vi "Selet PCBs.vi"(0 "data in":T11, 1 "Programming Data":T6, 5 "Dongle Fitted event Refnum in":T1, 7 "Edit VI":refnum<vi>, 11 "error in":errorcluster) -> (4 "data out":T11, 6 "Back":bool, 8 "Dongle fitted":bool, 15 "error out":errorcluster)   [LabVIEW 2013, in "Manipulate IPF.lvlib"]
uses:
  Manipulate IPF.lvlib
  3013/code/Modules/GUI/GUI_5/subPanels/edit/type_def/data.ctl
  3013/code/Modules/Configuration/type_def/Scan Params.ctl
  3013/code/Modules/Configuration/type_def/Profile Resolution.ctl
  3013/code/Modules/Preprocess Data/type_def/direction.ctl
  3013/code/Modules/Inspection/Data/Panel_class/type_def/Config File data.ctl
  3013/code/Modules/Inspection/type_def/Pos and Rot.ctl
  3013/code/Modules/Inspection/Data/PCB_class/type_def/PCB Params.ctl
  3013/code/Modules/Inspection/Data/Panel_class/type_def/BarCode Params.ctl
  3013/code/Modules/Barcode Reader/type_def/id.ctl
  3013/code/Modules/Inspection/Data/Panel_class/type_def/inspection data.ctl
  3013/code/Modules/Inspection/type_def/Range Limits.ctl
  type_def/but_back.ctl
  type_def/but_continue.ctl
  type_def/files.ctl
  type_def/PCB List.ctl
  type_def/Dongle fitted event refnum.ctl
  Pack Data/type_def/file types.ctl
  <vilib>/Utility/cursorutil.llb/Set Cursor (Icon Pict).vi
  3013/code/Modules/Barcode Reader/Barcode Reader.lvlib
  3013/code/Modules/Inspection/Inspection.lvlib
  3013/code/Modules/Inspection/Data/PCB_class/PCB.lvclass
  a3Di APG.lvlib
  3013/code/Modules/Inspection/Data/Panel_class/Panel.lvclass
  Pack Data/Pack Files.lvlib
  3013/code/Modules/Configuration/Config.lvlib
  3013/code/Modules/Preprocess Data/PreProcess.lvlib
  3013/code/Modules/GUI/GUI_5/subPanels/edit/edit.lvlib
panel:
  out "Within outline":bool
  out "XY":cluster{"X":dbl, "Y":dbl}
  out "PCB Name":string
  in  "PCB List":T2 {"gui"."PCB Params"."Pos & Rot"."Y" format="%#_8g"; "gui"."PCB Params"."Pos & Rot"."X" format="%#_8g"}
  out "XY Graph":cluster{"X Out":dbl[], "Y Out":dbl[]}[](graph)
  in  "Continue Button":T9
  in  "Back Button":T10
  # "Select PCBs"
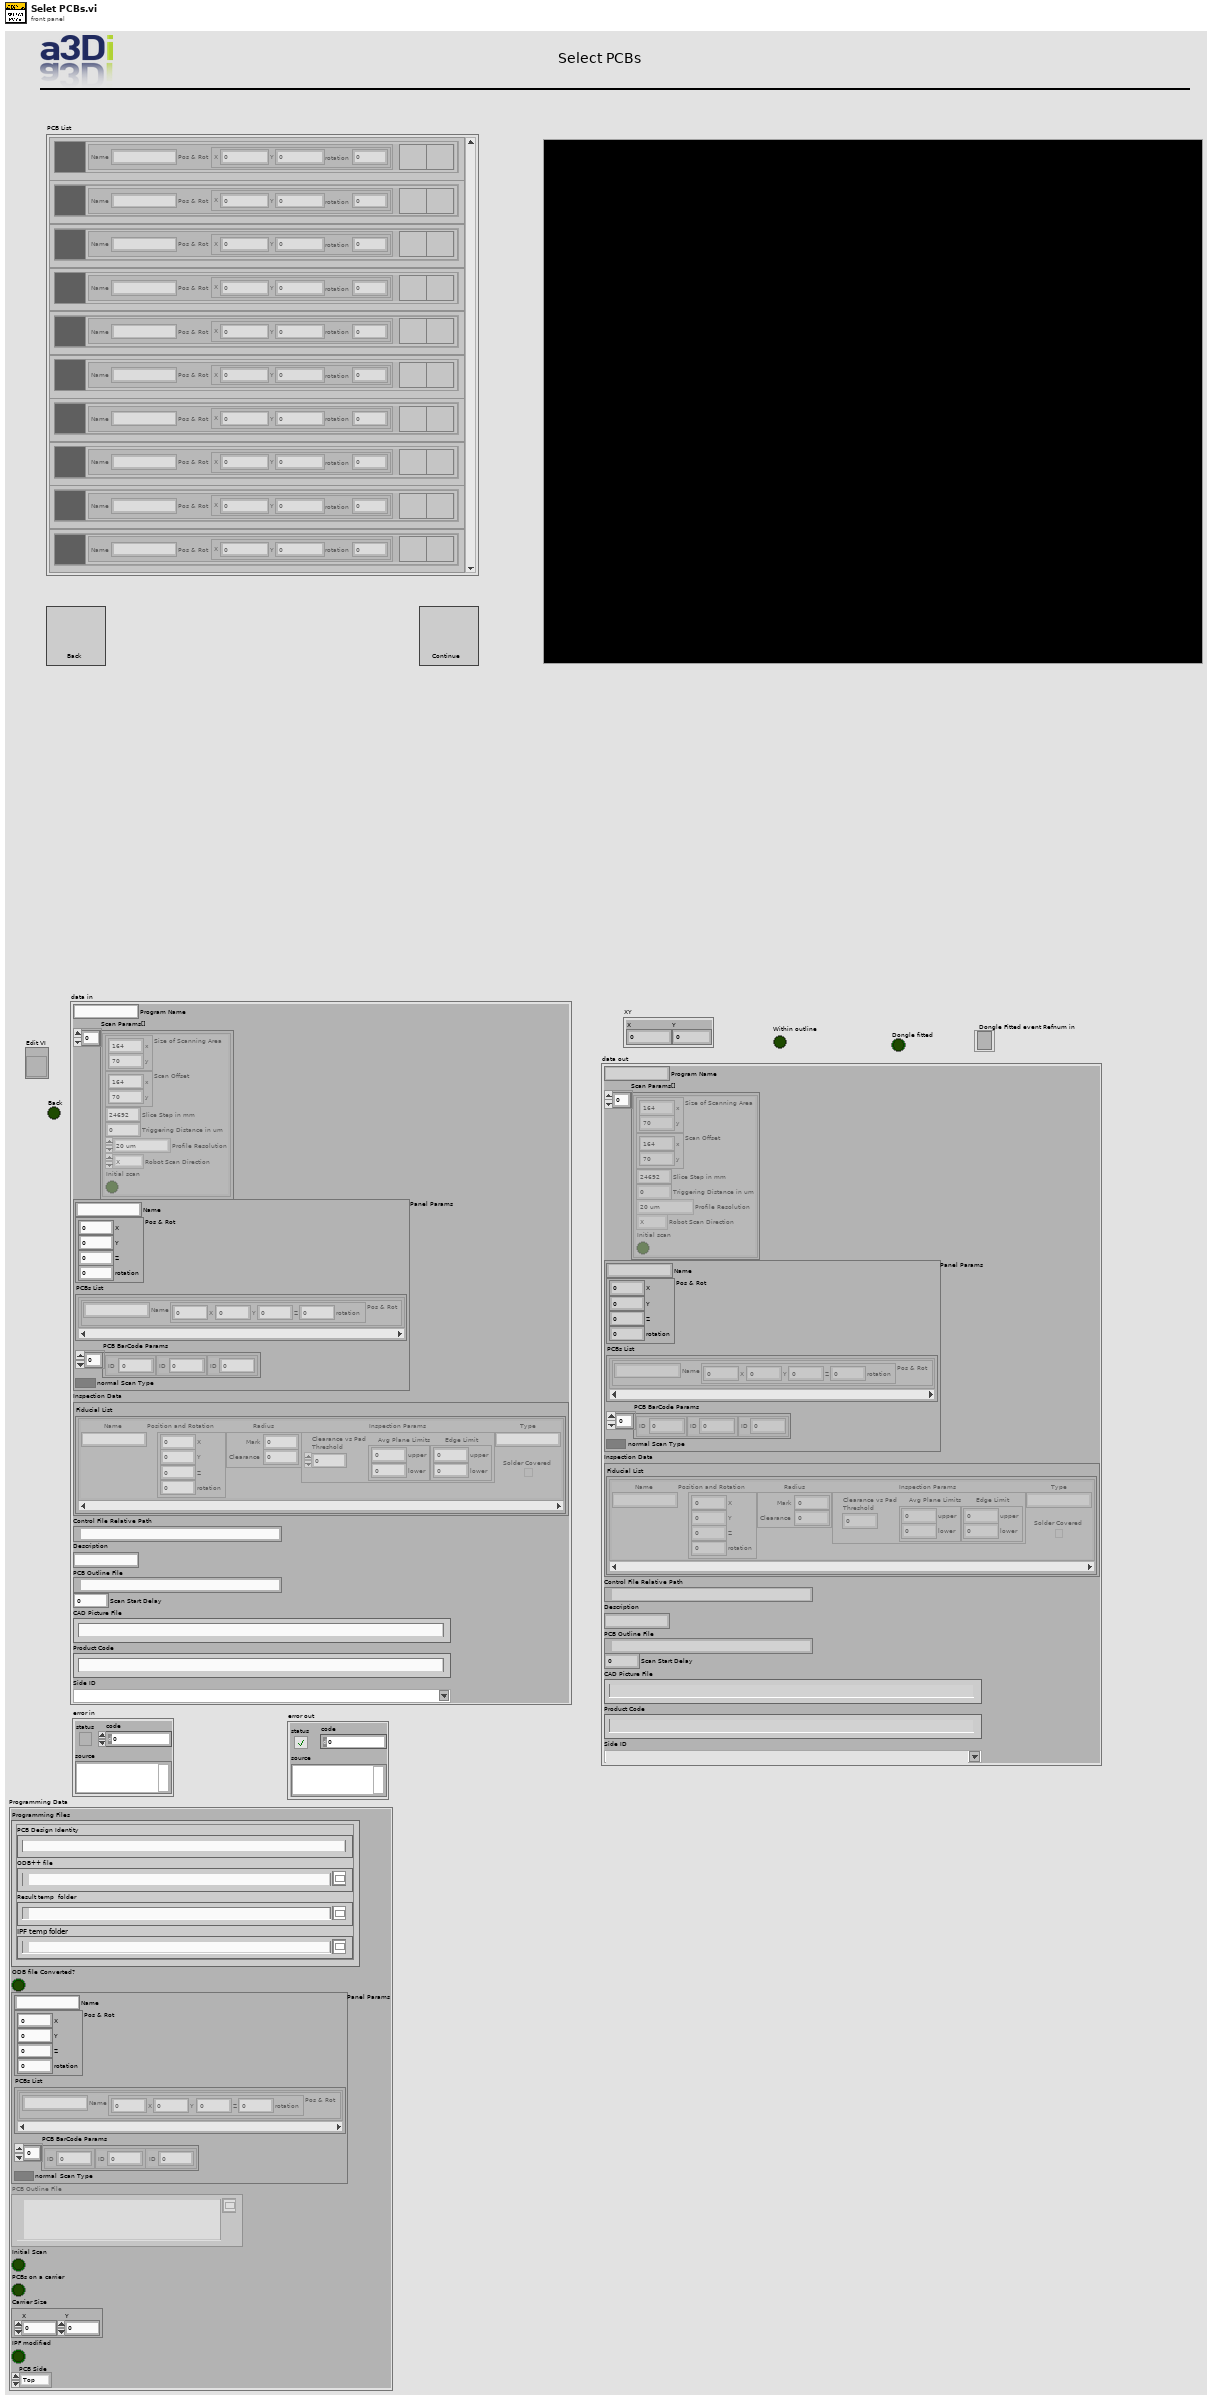
[diagram p1: front panel]
types:
  T1 = typedef "Dongle fitted event refnum.ctl" = refnum<event-registration>
  T2 = typedef "Manipulate IPF.lvlib/PCB List.ctl" = cluster{"Color Box":u32, "gui":cluster{"PCB Params":T3, "Barcode\nReader":cluster{"ID":T5}, "insert":bool, "delete":bool}}[]
  T3 = typedef "Inspection.lvlib/PCB.lvclass/PCB Params.ctl" = cluster{"Name":string, "Pos & Rot":T4}
  T4 = typedef "Inspection.lvlib/Pos and Rot.ctl" = cluster{"X":dbl, "Y":dbl, "Z":dbl, "rotation":dbl}
  T5 = typedef "Barcode Reader.lvlib/id.ctl" = u8
  T6 = typedef "a3Di APG.lvlib/files.ctl" = cluster{"Programming Files":cluster{"PCB Design Identity":string, "ODB++ file":path, "Result temp  folder":path, "IPF temp folder":path}, "ODB file Converted?":bool, "Panel Params":T7, "PCB Outline File":path, "Initial Scan":bool, "PCBs on a carrier":bool, "Carrier Size":cluster{"X":dbl, "Y":dbl}, "IPF modified":bool, "PCB Side":enum16{"Top", "Bottom"}}
  T7 = typedef "Inspection.lvlib/Panel.lvclass/Config File data.ctl" = cluster{"Name":string, "Pos & Rot":T4, "PCBs List":cluster{"PCB Params":T3}[], "PCB BarCode Params":T8[], "Scan Type":bool}
  T8 = typedef "Inspection.lvlib/Panel.lvclass/BarCode Params.ctl" = cluster{"ID":T5}
  T9 = typedef "but_continue.ctl" = bool
  T10 = typedef "a3Di APG.lvlib/but_back.ctl" = bool
  T11 = typedef "GUI.lvlib/subPanel.lvlib/edit.lvlib/data.ctl" = cluster{"Program Name":string, "Scan Params[]":T12[], "Panel Params":T7, "Inspection Data":T15, "Control File Relative Path":path, "Description":string, "PCB Outline File":path, "Scan Start Delay":dbl, "CAD Picture File":string, "Product Code":string, "Side ID":string}
  T12 = typedef "Config.lvlib/Scan Params.ctl" = cluster{"Size of Scanning Area":cluster{"x":dbl, "y":dbl}, "Scan Offset":cluster{"x":dbl, "y":dbl}, "Slice Step in mm":dbl, "Triggering Distance in mm":dbl, "Triggering Distance in um":dbl, "Profile Resolution":T13, "Version":string, "Robot Scan Direction":T14, "Initial scan":bool}
  T13 = typedef "Config.lvlib/Profile Resolution.ctl" = enum8{"20 um", "40 um"}
  T14 = typedef "PreProcess.lvlib/direction.ctl" = enum8{"X", "Y"}
  T15 = typedef "Inspection.lvlib/Panel.lvclass/inspection data.ctl" = cluster{"Fiducial List":cluster{"Name":string, "Position and Rotation":T4, "Radius":cluster{"Mark":dbl, "Clearance":dbl}, "Inspection Params":cluster{"Clearance vs Pad\nThreshold":dbl, "Avg Plane Limits":T16, "Edge Limit":T16}, "Type":string, "Solder Covered":bool}[]}
  T16 = typedef "Inspection.lvlib/Range Limits.ctl" = cluster{"upper":sgl, "lower":sgl}
  T17 = enum16{"Initialisaion", "Wait for user input", "exit"}
  T18 = cluster{"Plot colour":u32, "gui":cluster{"PCB Params":T3, "Barcode\nReader":cluster{"ID":T5}, "insert":bool, "delete":bool}}
  T19 = enum32{"Invalid", "Standard", "Closed", "Hidden", "Minimized", "Maximized"}
  T20 = typedef "Pack Files.lvlib/file types.ctl" = enum16{"ODB", "TCF", "CAD Outline", "Config", "Inspection Prog", "a3Di-bin", "Results", "CAD Labels", "CAD Pads", "calScan_fid", "calScan_cal-tab", "PCB_SerialNumber", "CAD_Assembly", "Version", "Old Results", "CAD Picture", "Old TCF"}
  T21 = enum8{"Enabled", "Disabled", "Disabled and Grayed Out"}
  T22 = cluster{"Plot colour":u32, "gui":cluster{"PCB Params":T3, "Barcode\nReader":cluster{"ID":T5}, "insert":bool, "delete":bool}}[]
  T23 = cluster{"Data":cluster{"X Out":dbl[], "Y Out":dbl[]}, "Name":string}[]
  T24 = cluster{"Color Box":bool, "gui":cluster{"PCB Params":cluster{"Name":bool, "Pos & Rot":cluster{"X":bool, "Y":bool, "Z":bool, "rotation":bool}}, "Barcode\nReader":cluster{"ID":bool}, "insert":bool, "delete":bool}}[]
  T25 = cluster{"Color Box":u32, "gui":cluster{"PCB Params":T3, "Barcode\nReader":cluster{"ID":T5}, "insert":bool, "delete":bool}}
  T26 = typedef "LVPoint32TypeDef.ctl" = cluster{"Horizontal":i32, "Vertical":i32}
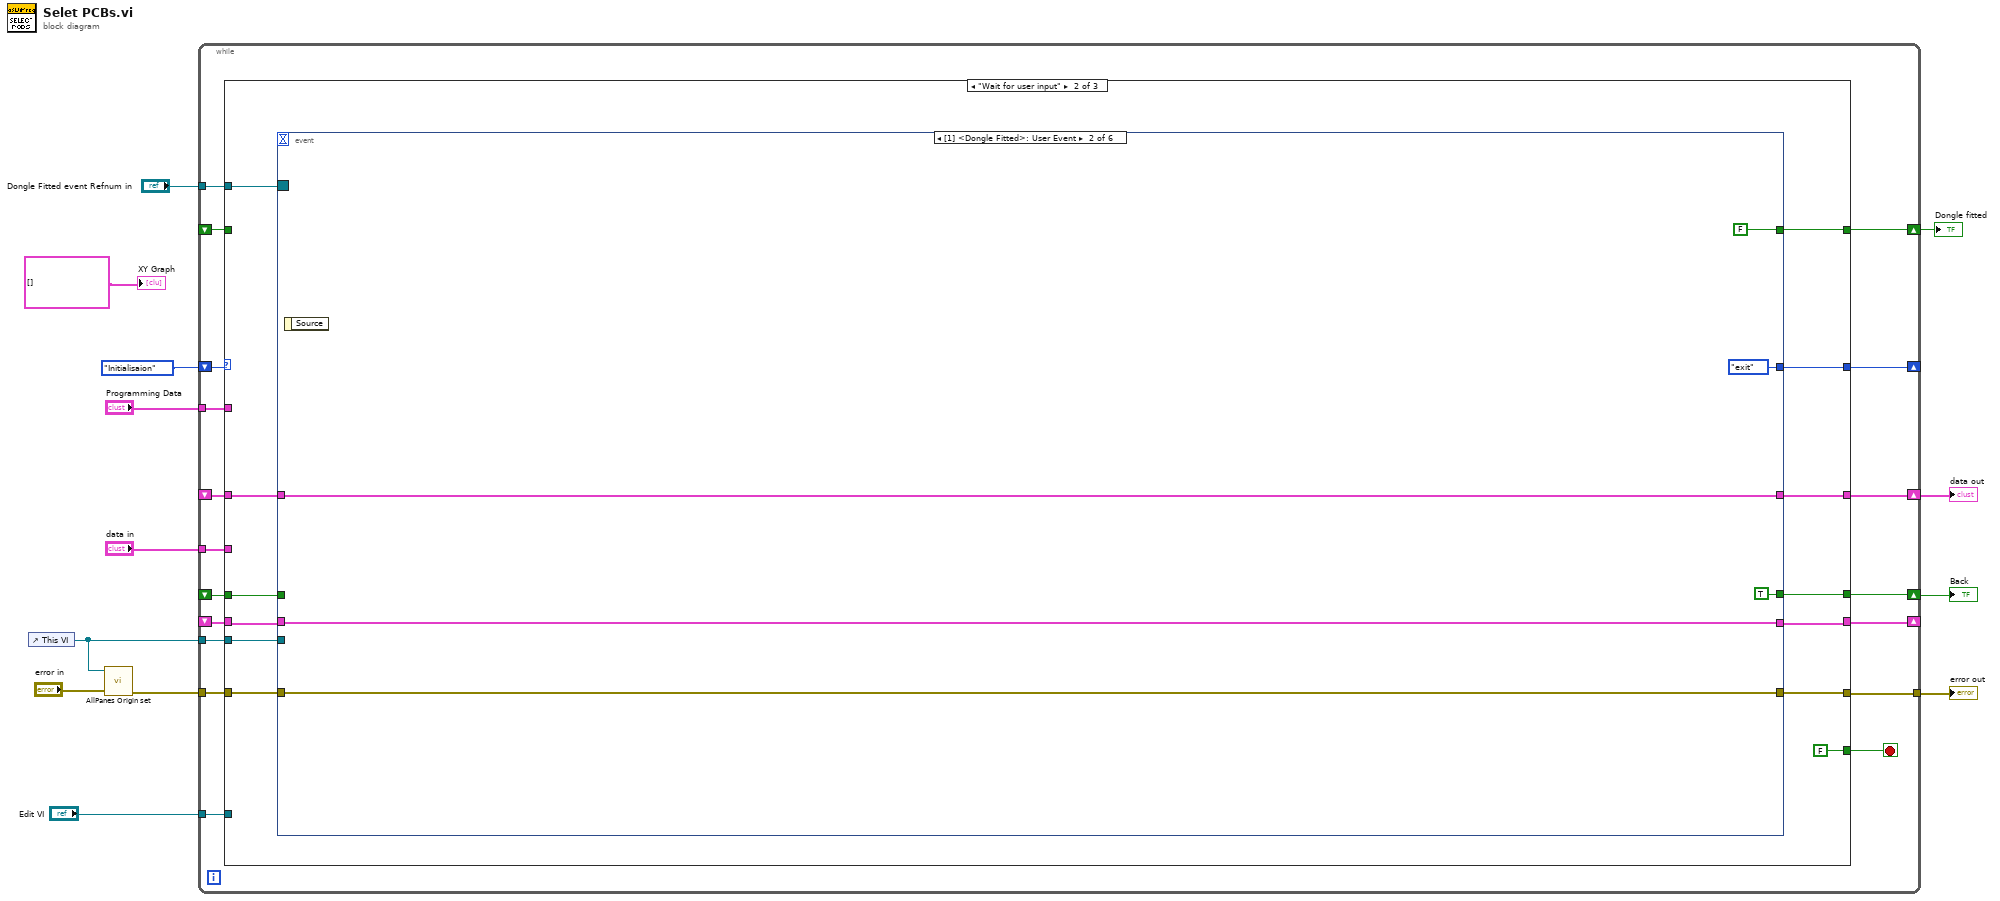
[diagram p0: block diagram]
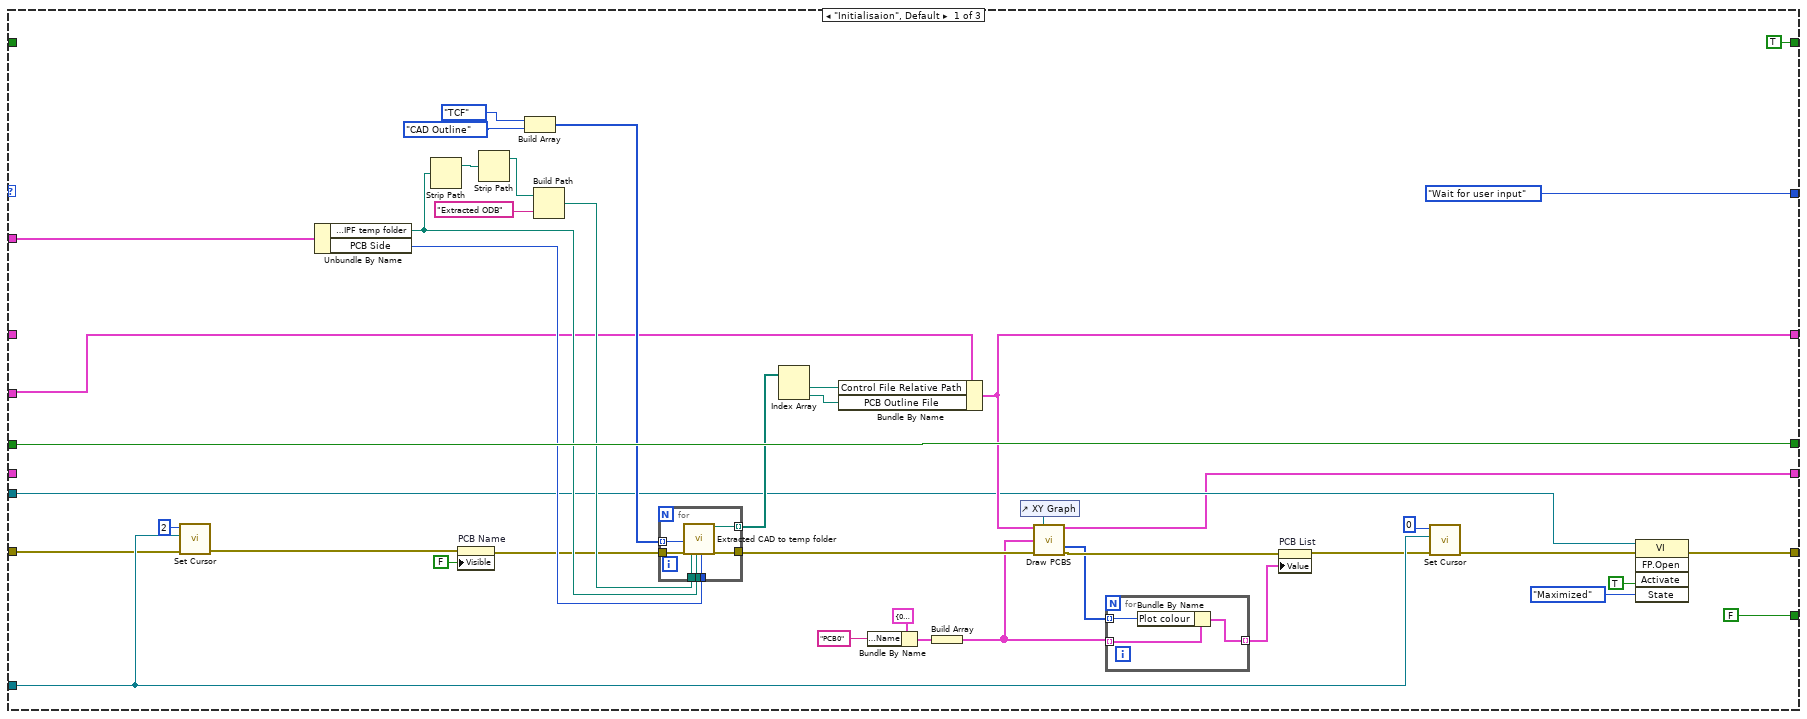
[diagram p2: hidden frame]
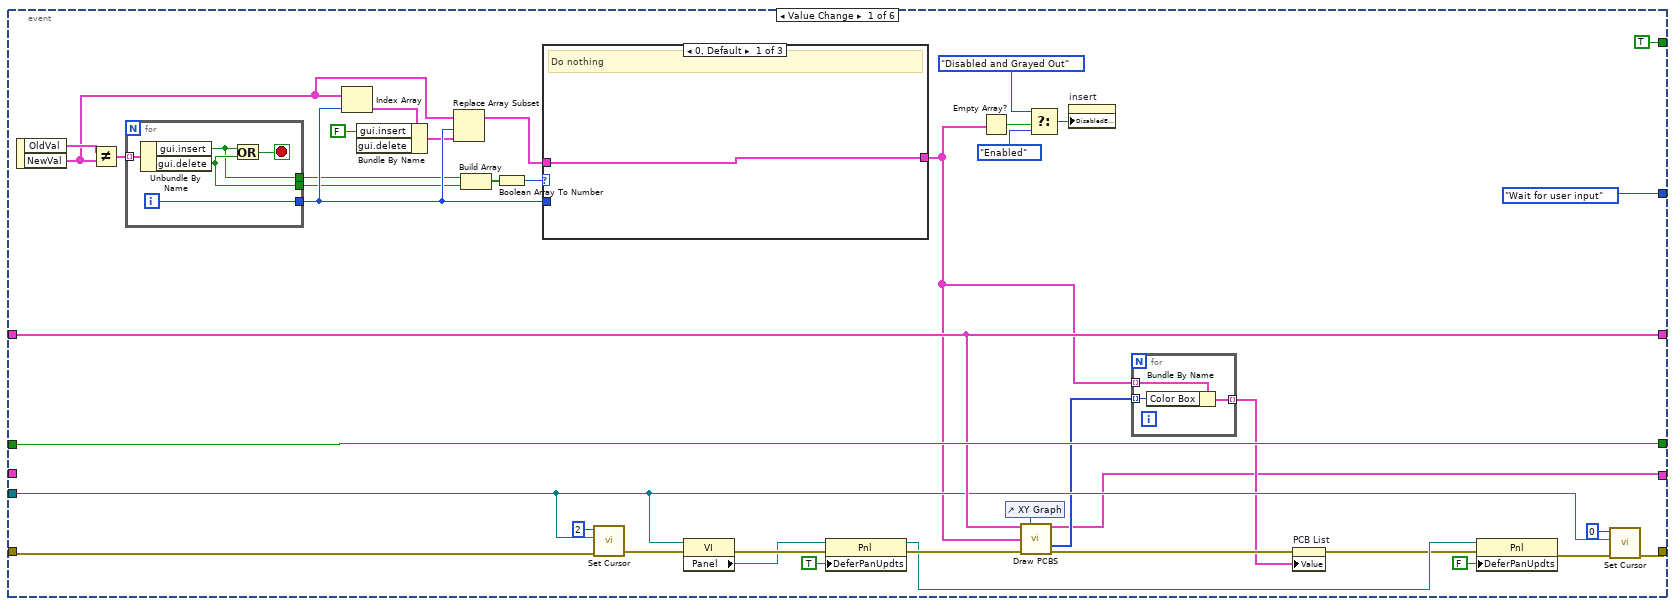
[diagram p3: hidden frame]
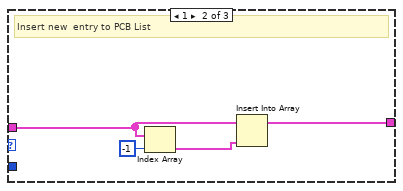
[diagram p4: hidden frame]
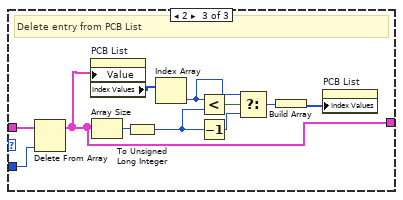
[diagram p5: hidden frame]
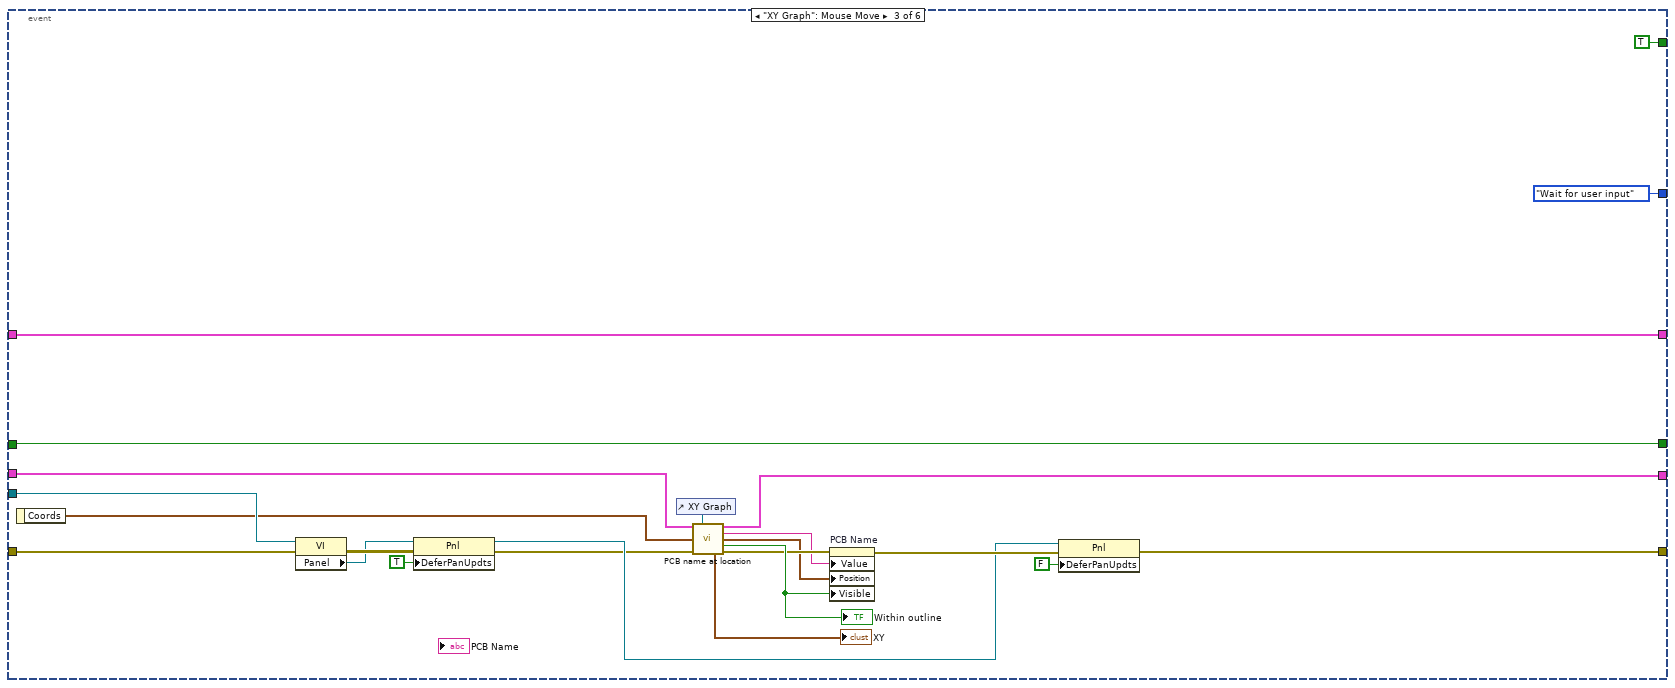
[diagram p6: hidden frame]
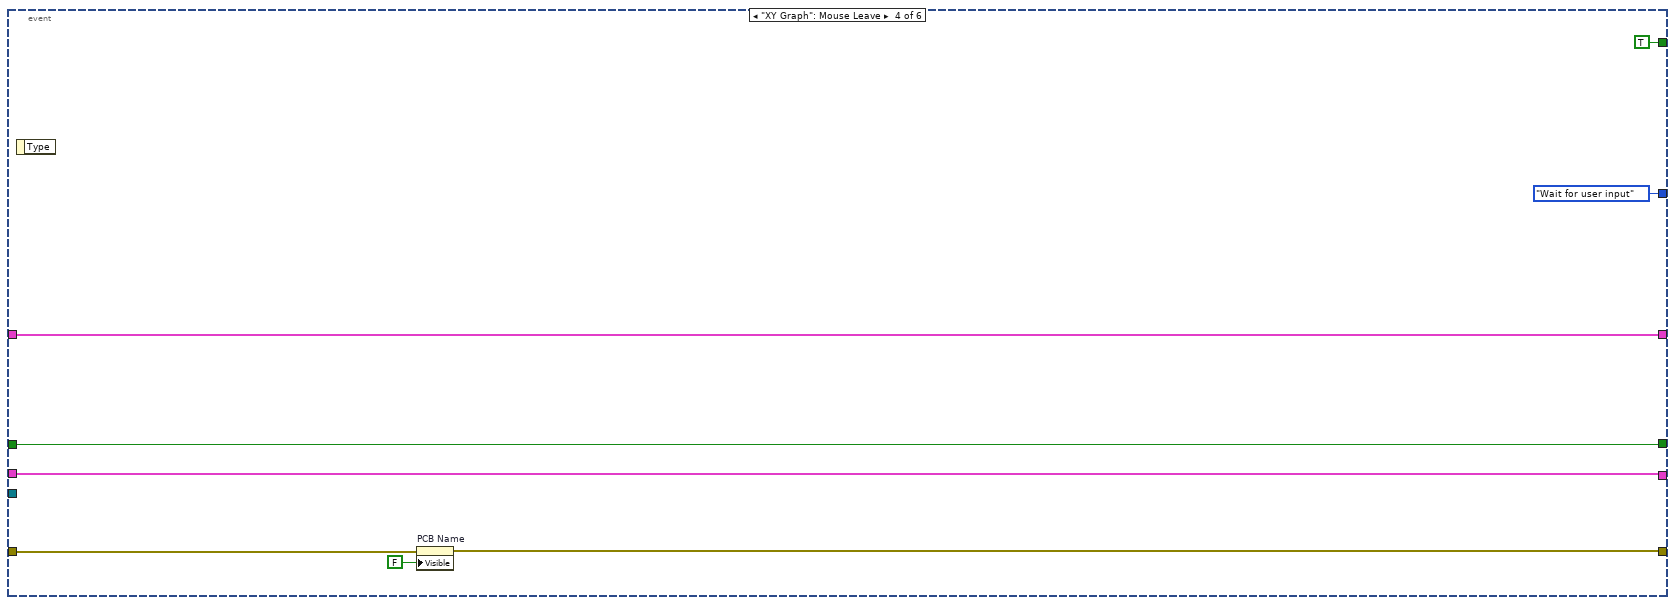
[diagram p7: hidden frame]
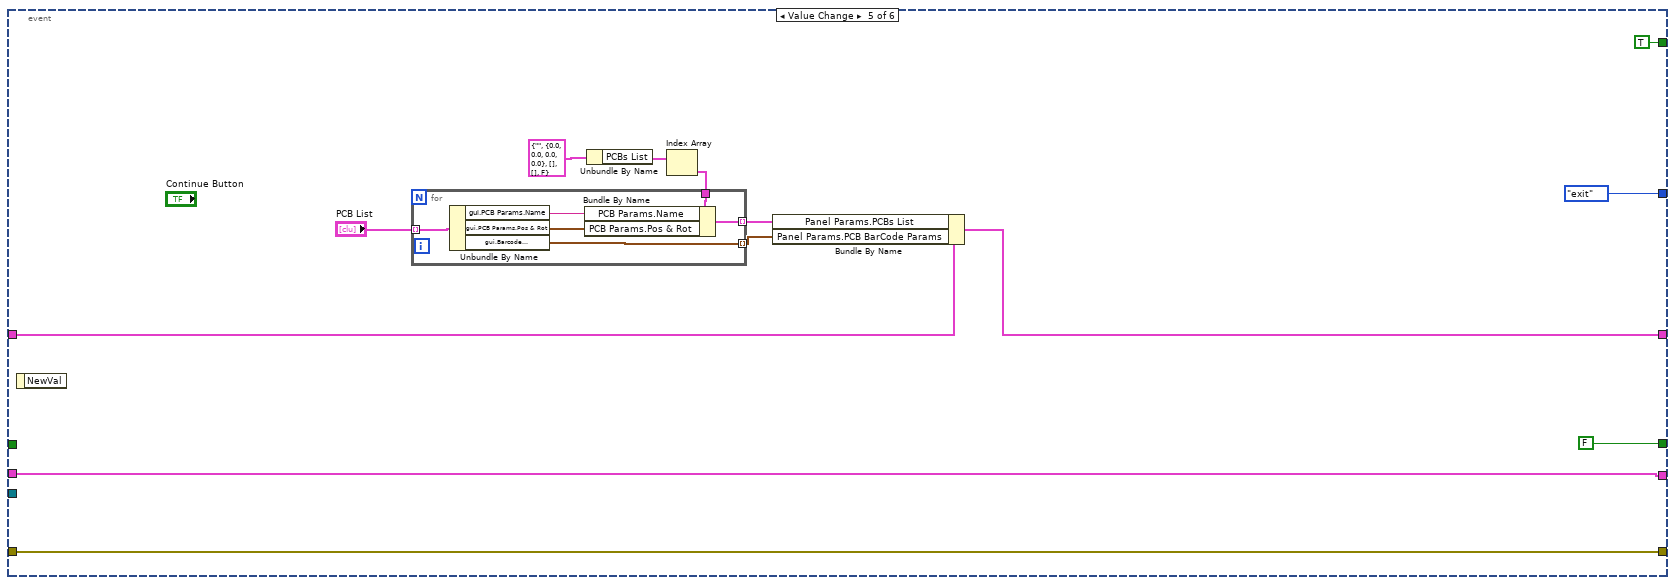
[diagram p8: hidden frame]
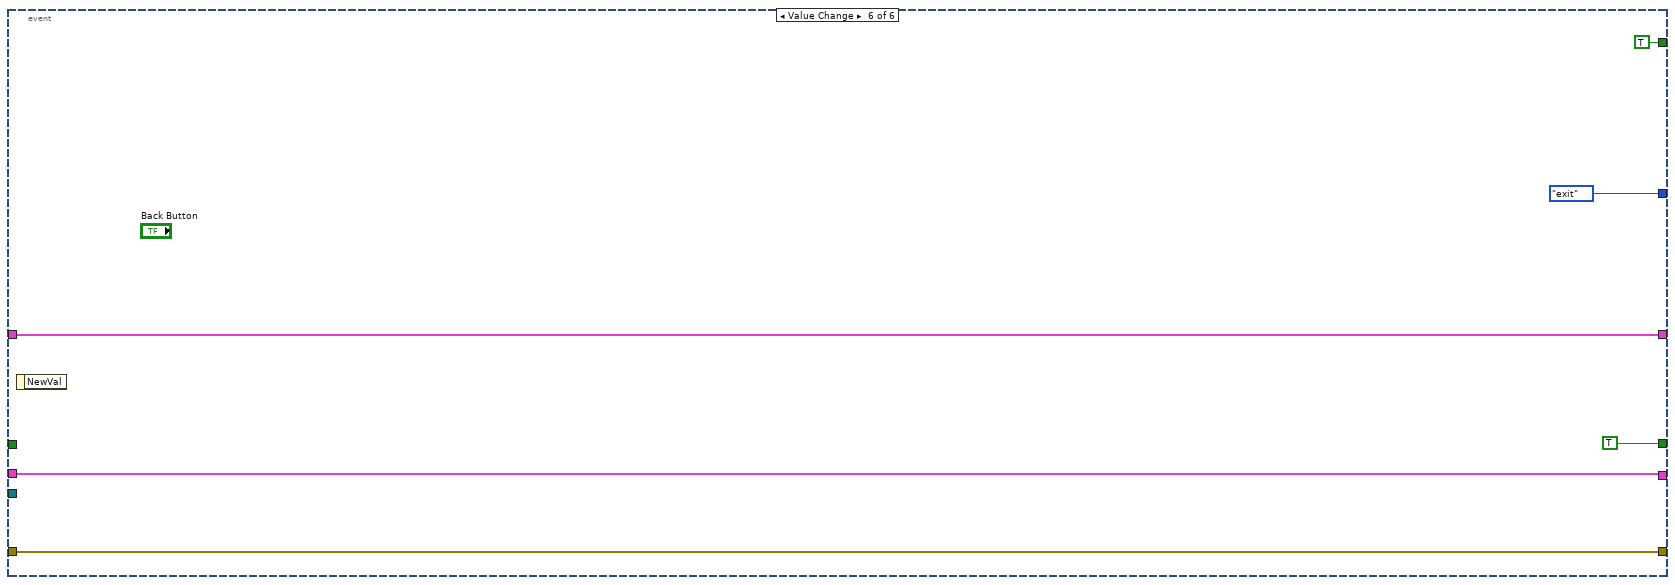
[diagram p9: hidden frame]
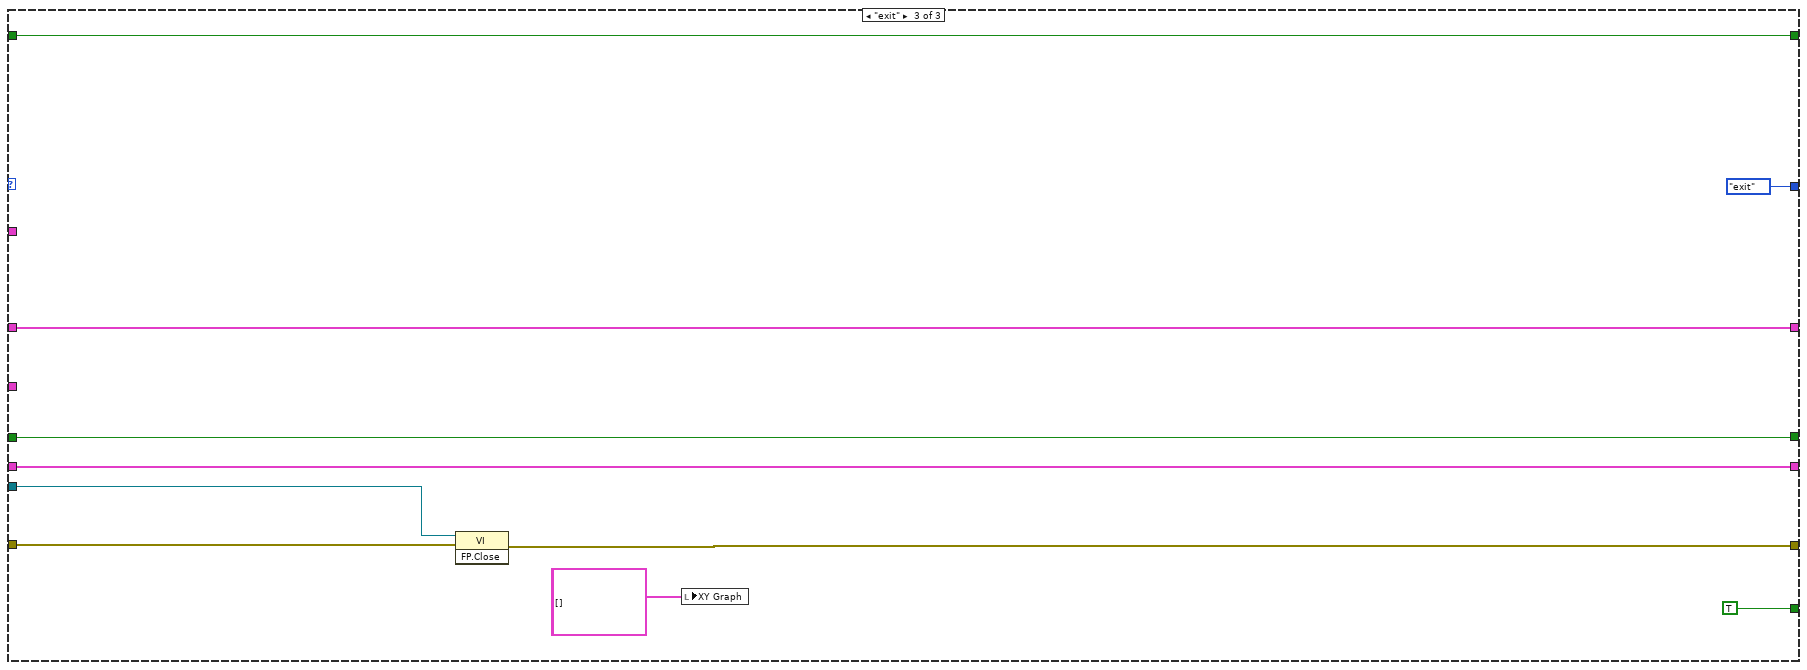
[diagram p10: hidden frame]
diagram:
  n1 = control-ref of="This VI"() -> (w9:refnum<vi>)
  n2 = call "AllPanes Origin set.vi"("VI ref in"=w9, "error in"="error in") -> ("error out"=w10:errorcluster)  [unwired: 12 in, 1 out]
  n3 = while {
    shift-right: [w29] -> _
    shift-left: T17."Initialisaion" -> [w31]
    tunnel: "data in" -> [w28]
    tunnel: w10 -> [w27]
    tunnel: w9 -> [w26]
    tunnel: [w25] -> w8
    shift-right: [w24] -> w7
    shift-left: _ -> [w23]
    shift-right: [w22] -> w6
    shift-left: _ -> [w21]
    tunnel: "Programming Data" -> [w20]
    tunnel: "Edit VI" -> [w19]
    shift-right: [w18] -> _
    shift-left: _ -> [w17]
    tunnel: "Dongle Fitted event Refnum in" -> [w16]
    shift-right: [w15] -> w1
    shift-left: _ -> [w14]
    stop <- w30 stop-if-true
    n4 = case shown="\"Wait for user input\"" w31 {
      tunnel: [FALSE FALSE TRUE] -> w30
      tunnel: [T17."Wait for user input" w95 T17."exit"] -> w29
      tunnel: w28 -> [w60 _ _]
      tunnel: w27 -> [w33 w94 w227]
      tunnel: w26 -> [w45 w88 w230]
      tunnel: [w46 w93 w226] -> w25
      tunnel: [w59 w91 w229] -> w24
      tunnel: w23 -> [_ w92 w229]
      tunnel: [w71 w90 w228] -> w22
      tunnel: w21 -> [w71 w89 w228]
      tunnel: w20 -> [w70 _ _]
      tunnel: w19 -> [w51 _ _]
      tunnel: [w38 w86 w224] -> w18
      tunnel: w17 -> [_ w87 w224]
      tunnel: w16 -> [_ w85 _]
      tunnel: [TRUE w84 w223] -> w15
      tunnel: w14 -> [_ _ w223]
      frame "Initialisaion", Default {
        n5 = call-poly <vilib>:"Set Cursor.vi"("error in (no error)"=w33, "VI reference (current VI)"=w51, "icon"=u16 2) -> ("error out"=w41:errorcluster)  [unwired: 7 in, 1 out]
        n6 = Unbundle By Name(w70) -> ("Programming Files.IPF temp folder"=w63:path, "PCB Side"=w69:enum16{"Top", "Bottom"})
        n7 = Strip Path(path=w63) -> (stripped path=w65:path)  [unwired: 1 out]
        n8 = property on="PCB Name" class="Str"(error in=w41, "Visible"=FALSE) -> (error out=w40:errorcluster)  [unwired: 1 in, 1 out]
        n9 = Strip Path(path=w65) -> (stripped path=w62:path)  [unwired: 1 out]
        n10 = Build Array(file_types."TCF" ("Descriptions"), file_types."CAD Outline" ("element")) -> (w66:T20[])
        n11 = Build Path(base path=w62, name or relative path="Extracted ODB") -> (appended path=w61:path)
        n12 = for {
          tunnel: [w83] -> w52
          tunnel: w69 -> [w82]
          tunnel: w63 -> [w81]
          tunnel: w66 -> [w80] mode=indexing
          tunnel: w61 -> [w79]
          tunnel: w40 -> [w78]
          tunnel: [w77] -> w58 mode=indexing
          n13 = call "Extracted CAD to temp folder.vi"("Descriptions"=w80, "error in (no error)"=w78, "Extracted ODB"=w79, "IPF temp folder"=w81, "PCB Side"=w82) -> ("Temp file path"=w77:path, "error out"=w83:errorcluster)  [unwired: 13 in]
        }
        n14 = Index Array(array=w58) -> (element #1=w57:path, element #2=w56:path)  [unwired: 2 in]
        n15 = Bundle By Name(cluster=w60, "Control File Relative Path"=w57, "PCB Outline File"=w56) -> (w59:T11)
        n16 = Bundle By Name(cluster=T18 {"Plot colour"=0, "gui"={"PCB Params"={"Name"="", "Pos & Rot"={"X"=0.0, "Y"=0.0, "Z"=0.0, "rotation"=0.0}}, "Barcode\nReader"={"ID"=0}, "insert"=FALSE, "delete"=FALSE}} ("PCB List"), "gui.PCB Params.Name"="PCB0" ("format string")) -> (w36:T18)
        n17 = Build Array(w36) -> (w35:T22)
        n18 = control-ref of="XY Graph"() -> (w55:refnum<vi>)
        n19 = call "Draw PCBS.vi"("data in"=w59, "XY Graph"=w55, "PCB List"=w35, "error in (no error)"=w52) -> ("PCB Outlines"=w38:T23, "Plot colours[]"=w42:u32[], "error out"=w50:errorcluster)  [unwired: 9 in]
        n20 = for {
          tunnel: w35 -> [w76] mode=indexing
          tunnel: [w75] -> w49 mode=indexing
          tunnel: w42 -> [w74] mode=indexing
          n21 = Bundle By Name(cluster=w76, "Plot colour"=w74) -> (w75:T18)
        }
        n22 = property on="PCB List" class="Arr"(error in=w50, "Value"=w49) -> (error out=w48:errorcluster)  [unwired: 1 in, 1 out]
        n23 = call-poly <vilib>:"Set Cursor.vi"("error in (no error)"=w48, "VI reference (current VI)"=w51, "icon"=u16 0) -> ("error out"=w47:errorcluster)  [unwired: 7 in, 1 out]
        n24 = invoke class="VI" method="FP.Open"(reference=w45, error in=w47, "Activate"=TRUE ("Activate?"), "State"=T19."Maximized") -> (error out=w46:errorcluster)  [unwired: 1 in, 4 out]
      }
      frame "Wait for user input" {
        n25 = event shown="[1] <Dongle Fitted>: User Event" {
          selector: w85 -> [_ _ _ _ _ _]
          dyn-events: _ -> [_ _ _ _ _ _]
          timeout: _ -> [_ _ _ _ _ _]
          tunnel: [T17."Wait for user input" T17."exit" T17."Wait for user input" T17."Wait for user input" T17."exit" T17."exit"] -> w95
          tunnel: w94 -> [w112 w166 w178 w192 w209 w221]
          tunnel: [w107 w166 w185 w191 w209 w221] -> w93
          tunnel: w92 -> [w117 w163 w188 w195 w203 w222]
          tunnel: [w117 w163 w188 w195 w204 w222] -> w91
          tunnel: [w119 TRUE ("NewVal") w187 w197 FALSE ("NewVal") TRUE ("NewVal")] -> w90
          tunnel: w89 -> [w119 _ w187 w197 _ _]
          tunnel: w88 -> [w106 _ w183 _ _ _]
          tunnel: w87 -> [_ w165 w182 w193 w199 w218]
          tunnel: [w98 w165 w181 w193 w199 w218] -> w86
          tunnel: [TRUE FALSE TRUE TRUE TRUE TRUE] -> w84
          event Value Change {
            w126 = FALSE ("insert")
            n26 = event-data() -> ("OldVal"=w125:T2, "NewVal"=w124:T2)  [unwired: 1 in]
            n27 = Not Equal?(x=w125, y=w124) -> (x != y?=w132:T24)
            n28 = for {
              tunnel: w132 -> [w158] mode=indexing
              tunnel: [w157] -> w131
              tunnel: [w159] -> w130
              tunnel: [w160] -> w135
              i -> [w160]
              stop <- w156 stop-if-true
              n29 = Unbundle By Name(w158) -> ("gui.insert"=w157:bool, "gui.delete"=w159:bool)
              n30 = Or(x=w157, y=w159) -> (x .or. y?=w156:bool)
            }
            n31 = Index Array(array=w124, index=w135) -> (element=w128:T25)
            n32 = Bundle By Name(cluster=w128, "gui.insert"=w126, "gui.delete"=w126) -> (w127:T25)
            n33 = Replace Array Subset(array=w124, new element=w127, index=w135) -> (w133:T2)
            n34 = Build Array(w131, w130) -> (w129:bool[])
            n35 = Boolean Array To Number(Boolean array=w129) -> (number=w134:u32)
            n36 = case shown="0, Default" w134 {
              tunnel: w135 -> [_ _ w145]
              tunnel: [w140 w144 w149] -> w99
              tunnel: w133 -> [w140 w143 w155]
              frame 0, Default {
                # "Do nothing"
              }
              frame 1 {
                # "Insert new  entry to PCB List"
                n37 = Index Array(array=w143, index=-1) -> (element=w141:T25)
                n38 = Insert Into Array(array=w143, new element=w141) -> (w144:T2)  [unwired: 1 in]
              }
              frame 2 {
                # "Delete entry from PCB List"
                n39 = Delete From Array(array=w155, index=w145) -> (array with subset deleted=w149:T2)  [unwired: 1 in, 1 out]
                n40 = property on="PCB List" class="Arr"("Value"=w149) -> ("Index Values"=w148:u32[])  [unwired: 2 in, 2 out]
                n41 = Array Size(array=w149) -> (size(s)=w153:i32)
                n42 = To Unsigned Long Integer(number=w153) -> (unsigned 32bit integer=w151:u32)
                n43 = Index Array(array=w148) -> (element=w147:u32)  [unwired: 1 in]
                n44 = Less?(x=w147, y=w151) -> (x < y?=w152:bool)
                n45 = Decrement(x=w151) -> (x-1=w150:u32)
                n46 = Select(t=w147, s=w152, f=w150) -> (s? t:f=w154:u32)
                n47 = Build Array(w154) -> (w146:u32[])
                n48 = property on="PCB List" class="Arr"("Index Values"=w146) -> ()  [unwired: 2 in, 2 out]
              }
            }
            n49 = call-poly <vilib>:"Set Cursor.vi"("error in (no error)"=w112, "VI reference (current VI)"=w106, "icon"=u16 2) -> ("error out"=w111:errorcluster)  [unwired: 7 in, 1 out]
            n50 = property class="VI"(reference=w106, error in=w111) -> (error out=w116:errorcluster, "Panel"=w105:refnum<vi>)  [unwired: 1 out]
            n51 = property class="Pnl"(reference=w105, error in=w116, "DeferPanUpdts"=TRUE ("Defer Panel Updates")) -> (reference out=w104:refnum<vi>, error out=w113:errorcluster)
            n52 = Empty Array?(array=w99) -> (empty?=w122:bool)
            n53 = control-ref of="XY Graph"() -> (w118:refnum<vi>)
            n54 = call "Draw PCBS.vi"("data in"=w117, "XY Graph"=w118, "PCB List"=w99, "error in (no error)"=w113) -> ("PCB Outlines"=w98:T23, "Plot colours[]"=w100:u32[], "error out"=w102:errorcluster)  [unwired: 9 in]
            n55 = Select(t=T21."Disabled and Grayed Out" ("Disabled"), s=w122, f=T21."Enabled" ("Disabled")) -> (s? t:f=w123:T21)
            n56 = property on="insert" class="Bool"("DisabledEnum"=w123) -> ()  [unwired: 2 in, 2 out]
            n57 = for {
              tunnel: w99 -> [w139] mode=indexing
              tunnel: [w138] -> w101 mode=indexing
              tunnel: w100 -> [w137] mode=indexing
              n58 = Bundle By Name(cluster=w139, "Color Box"=w137) -> (w138:T25)
            }
            n59 = property on="PCB List" class="Arr"(error in=w102, "Value"=w101) -> (error out=w103:errorcluster)  [unwired: 1 in, 1 out]
            n60 = property class="Pnl"(reference=w104, error in=w103, "DeferPanUpdts"=FALSE ("Defer Panel Updates")) -> (error out=w108:errorcluster)  [unwired: 1 out]
            n61 = call-poly <vilib>:"Set Cursor.vi"("error in (no error)"=w108, "VI reference (current VI)"=w106, "icon"=u16 0) -> ("error out"=w107:errorcluster)  [unwired: 7 in, 1 out]
          }
          event User Event {
            n62 = event-data() -> ()  [unwired: 1 in, 1 out]
          }
          event "XY Graph": Mouse Move {
            n63 = event-data() -> ("Coords"=w177:T26)  [unwired: 1 in]
            n64 = property class="VI"(reference=w183, error in=w178) -> (error out=w171:errorcluster, "Panel"=w169:refnum<vi>)  [unwired: 1 out]
            n65 = property class="Pnl"(reference=w169, error in=w171, "DeferPanUpdts"=TRUE ("Defer Panel Updates")) -> (reference out=w184:refnum<vi>, error out=w175:errorcluster)
            n66 = control-ref of="XY Graph"() -> (w179:refnum<vi>)
            n67 = call "PCB name at location.vi"("PCB Outlines in"=w182, "XY Graph"=w179, "XY"=w177, "error in"=w175) -> ("PCB Outlines out"=w181:T23, "PCB Name"=w173:string, "Outline mean"=w172:cluster{"X":dbl, "Y":dbl}, "Within outline"=w180:bool, "x y position"=→"XY":cluster{"X":dbl, "Y":dbl}, "error out"=w174:errorcluster)  [unwired: 6 in]
            "Within outline" <- w180
            n68 = property on="PCB Name" class="Str"(error in=w174, "Value"=w173, "Position"=w172, "Visible"=w180) -> (error out=w186:errorcluster)  [unwired: 1 in, 1 out]
            n69 = property class="Pnl"(reference=w184, error in=w186, "DeferPanUpdts"=FALSE ("Defer Panel Updates")) -> (error out=w185:errorcluster)  [unwired: 1 out]
          }
          event "XY Graph": Mouse Leave {
            n70 = event-data() -> ()  [unwired: 1 in, 1 out]
            n71 = property on="PCB Name" class="Str"(error in=w192, "Visible"=FALSE) -> (error out=w191:errorcluster)  [unwired: 1 in, 1 out]
          }
          event Value Change {
            n72 = event-data() -> ()  [unwired: 1 in, 1 out]
            n73 = Unbundle By Name(T7 {"Name"="", "Pos & Rot"={"X"=0.0, "Y"=0.0, "Z"=0.0, "rotation"=0.0}, "PCBs List"=[], "PCB BarCode Params"=[], "Scan Type"=FALSE} ("Panel Params")) -> ("PCBs List"=w207:cluster{"PCB Params":T3}[])
            n74 = Index Array(array=w207) -> (element=w208:cluster{"PCB Params":T3})  [unwired: 1 in]
            n75 = for {
              tunnel: [w216] -> w205 mode=indexing
              tunnel: w208 -> [w215]
              tunnel: [w214] -> w201 mode=indexing
              tunnel: "PCB List" -> [w213] mode=indexing
              n76 = Unbundle By Name(w213) -> ("gui.PCB Params.Name"=w212:string, "gui.PCB Params.Pos & Rot"=w211:T4, "gui.Barcode\nReader"=w214:cluster{"ID":T5})
              n77 = Bundle By Name(cluster=w215, "PCB Params.Name"=w212, "PCB Params.Pos & Rot"=w211) -> (w216:cluster{"PCB Params":T3})
            }
            n78 = Bundle By Name(cluster=w203, "Panel Params.PCBs List"=w205, "Panel Params.PCB BarCode Params"=w201) -> (w204:T11)
          }
          event Value Change {
            n79 = event-data() -> ()  [unwired: 1 in, 1 out]
          }
        }
      }
      frame "exit" {
        (unwired) cluster{"X Out":dbl[], "Y Out":dbl[]}[] [] ("XY Graph")
        n80 = invoke class="VI" method="FP.Close"(reference=w230, error in=w227) -> (error out=w226:errorcluster)  [unwired: 1 in, 2 out]
        n81 = local write "XY Graph"(cluster{"X Out":dbl[], "Y Out":dbl[]}[] [] ("XY Graph")) -> ()
      }
    }
  }
  "error out" <- w8
  "data out" <- w7
  "Back" <- w6
  "Dongle fitted" <- w1
  "XY Graph" <- cluster{"X Out":dbl[], "Y Out":dbl[]}[] [] ("XY Graph")
